vi "DFD IIR Comb Design.vi"   [LabVIEW 2017, in "NI_DigFilterLicensed.lvlib"]
doc: "Creates an infinite impulse response (IIR) comb filter. You must manually select the polymorphic instance you want to use."
uses:
  <vilib>/addons/Digital Filter Design/NI_DigFilterLicensed.lvlib
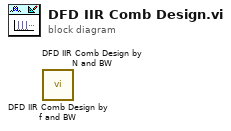
[diagram p0: block diagram]
diagram:
  n1 = call <vilib>:"DFD IIR Comb Design by f and BW.vi"() -> ()  [unwired: 10 in, 2 out]
  n2 = call <vilib>:"DFD IIR Comb Design by N and BW.vi"() -> ()  [unwired: 10 in, 2 out]
